vi "graph 2 .vi"() -> ()   [LabVIEW 2019]
panel:
  out "Waveform Graph":cluster{i32, dbl, dbl[]}(graph)
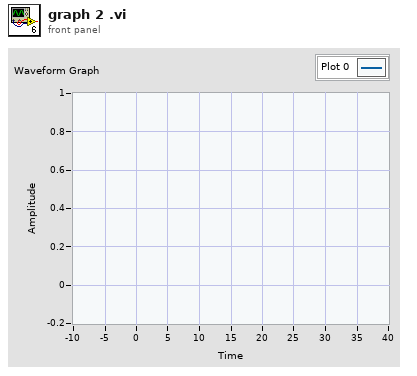
[diagram p1: front panel]
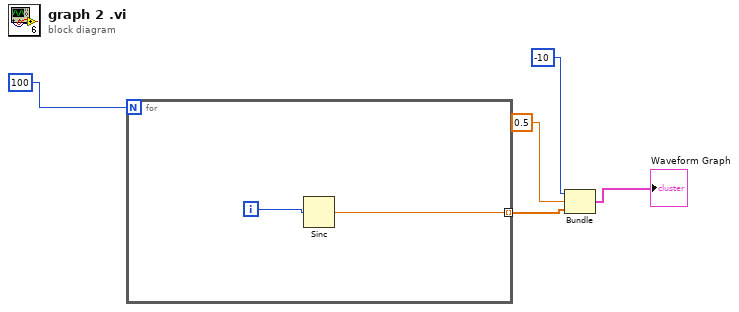
[diagram p0: block diagram]
diagram:
  n1 = for {
    N: 100 -> [_]
    tunnel: [w6] -> w2 mode=indexing
    i -> [w7]
    n2 = Sinc(1:w7) -> (0:w6:dbl)
  }
  n3 = Bundle(-10, 0.5, w2) -> (→"Waveform Graph":cluster{i32, dbl, dbl[]})  [unwired: 1 in]
